vi "toml_error.vi"(7 "message":string, 8 "error in (no error)":errorcluster, 10 "offset (0)":i32, 11 "toml":string) -> (0 "error out":errorcluster)   [LabVIEW 2017]
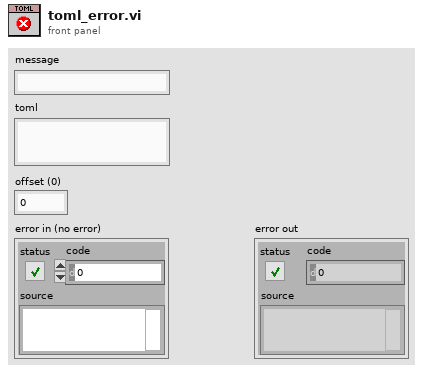
[diagram p1: front panel]
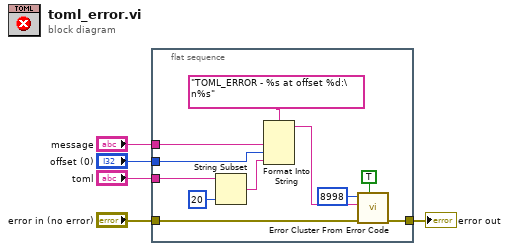
[diagram p0: block diagram]
diagram:
  n1 = flat-sequence {
    tunnel: "error in (no error)" -> [w16]
    tunnel: [w13] -> w4
    tunnel: "toml" -> [w12]
    tunnel: "message" -> [w10]
    tunnel: "offset (0)" -> [w9]
    frame #0 {
      n2 = String Subset(string=w12, length (rest)=20 ("length (rest)")) -> (substring=w7:string)  [unwired: 1 in]
      n3 = Format Into String(format string="TOML_ERROR - %s at offset %d:\n%s", w10, w9, w7) -> (resulting string=w6:string)  [unwired: 2 in, 1 out]
      n4 = call <vilib>:"Error Cluster From Error Code.vi"("show call chain? (False)"=TRUE, "error in (no error)"=w16, "error message (\"\")"=w6, "error code (0)"=8998) -> ("error out"=w13:errorcluster)  [unwired: 5 in]
    }
  }
  "error out" <- w4
